vi "Simulation Deployment Utility.vi"() -> ()   [LabVIEW 2020]
panel:
  in  "Password":string
  in  "Username":string
  in  "stop model":bool
  in  "start model":bool
  in  "Compiled model path":path
  out "Status":string
  in  "Target IP Address":string
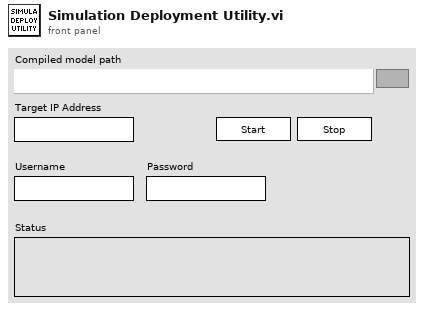
[diagram p1: front panel]
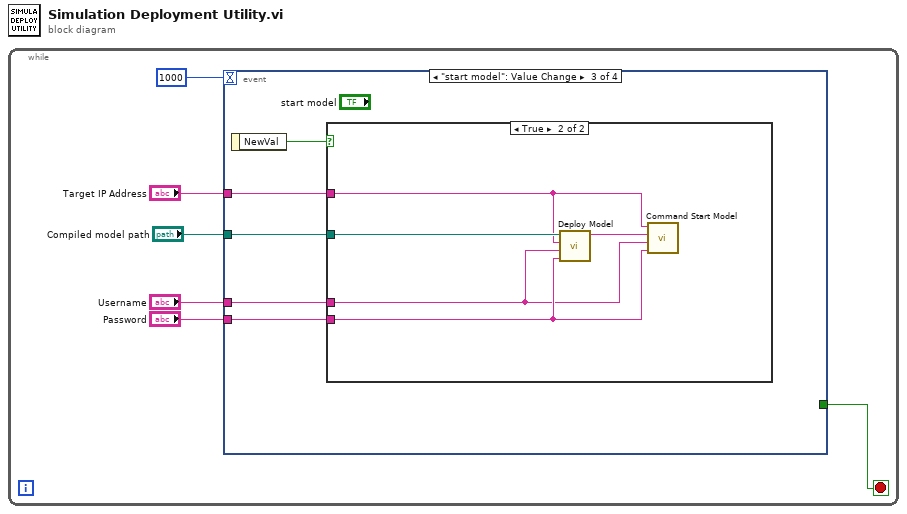
[diagram p0: block diagram]
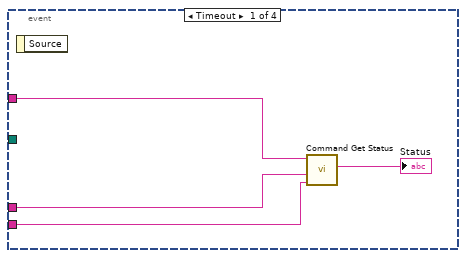
[diagram p2: hidden frame]
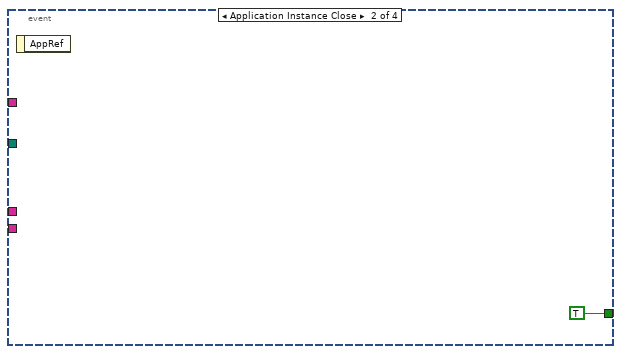
[diagram p3: hidden frame]
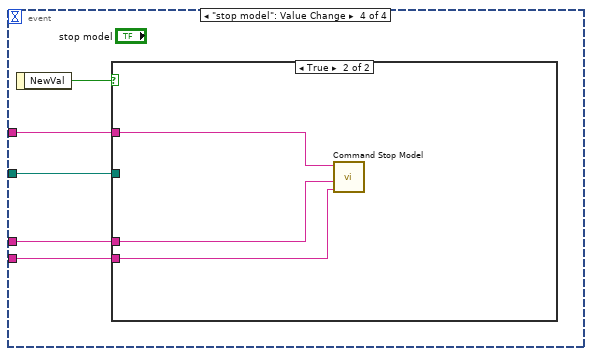
[diagram p5: hidden frame]
diagram:
  n1 = while {
    stop <- w1 stop-if-true
    n2 = event shown="[2] \"start model\": Value Change" {
      selector: _ -> [_ _ _ _]
      dyn-events: _ -> [_ _ _ _]
      timeout: 1000 -> [_ _ _ _]
      tunnel: "Compiled model path" -> [_ _ w15 w25]
      tunnel: "Target IP Address" -> [w10 _ w14 w24]
      tunnel: "Password" -> [w8 _ w13 w23]
      tunnel: "Username" -> [w9 _ w12 w22]
      tunnel: [_ TRUE _ _] -> w1
      event Timeout {
        n3 = event-data() -> ()  [unwired: 1 in, 1 out]
        n4 = call "Command Get Status.vi"("Password"=w8, "Username"=w9, "Target IP Address"=w10) -> ("Status"=→"Status":string)  [unwired: 7 in, 1 out]
      }
      event Application Instance Close {
        n5 = event-data() -> ()  [unwired: 1 in, 1 out]
      }
      event "start model": Value Change {
        n6 = event-data() -> ("NewVal"=w16:bool)  [unwired: 1 in]
        n7 = case shown="True" w16 {
          tunnel: w15 -> [_ w20]
          tunnel: w14 -> [_ w19]
          tunnel: w13 -> [_ w18]
          tunnel: w12 -> [_ w17]
          frame False {
          }
          frame True {
            n8 = call "Deploy Model.vi"("Password"=w18, "Username"=w17, "Target IP Address"=w19, "Local Model Path"=w20) -> ("Remote File Path"=w21:string)  [unwired: 6 in, 1 out]
            n9 = call "Command Start Model.vi"("Password"=w18, "Username"=w17, "Remote Model Path"=w21, "Target IP Address"=w19) -> ()  [unwired: 7 in, 1 out]
          }
        }
      }
      event "stop model": Value Change {
        n10 = event-data() -> ("NewVal"=w26:bool)  [unwired: 1 in]
        n11 = case shown="True" w26 {
          tunnel: w25 -> [_ _]
          tunnel: w24 -> [_ w29]
          tunnel: w23 -> [_ w28]
          tunnel: w22 -> [_ w27]
          frame False {
          }
          frame True {
            n12 = call "Command Stop Model.vi"("Password"=w28, "Username"=w27, "Target IP Address"=w29) -> ()  [unwired: 8 in, 1 out]
          }
        }
      }
    }
  }
